vi "Data Array Tag.vi"(8 "error in (no error)":errorcluster, 11 "Node Ptr":T1 format="%.0x") -> (0 "error out":errorcluster)   [LabVIEW 2015, in "OPC UA Client System Explorer.lvlib"]
uses:
  OPC UA Client System Explorer.lvlib
  <vilib>/NI Veristand/Custom Device API/Custom Device Item Ref.ctl
  <vilib>/NI Veristand/Custom Device API/Custom Device API.lvlib
panel:
  out "Name":string
  in  "Header":cluster{"Section Name":string}={"Section Name"="Data Tag Settings"}
  in  "Description":string
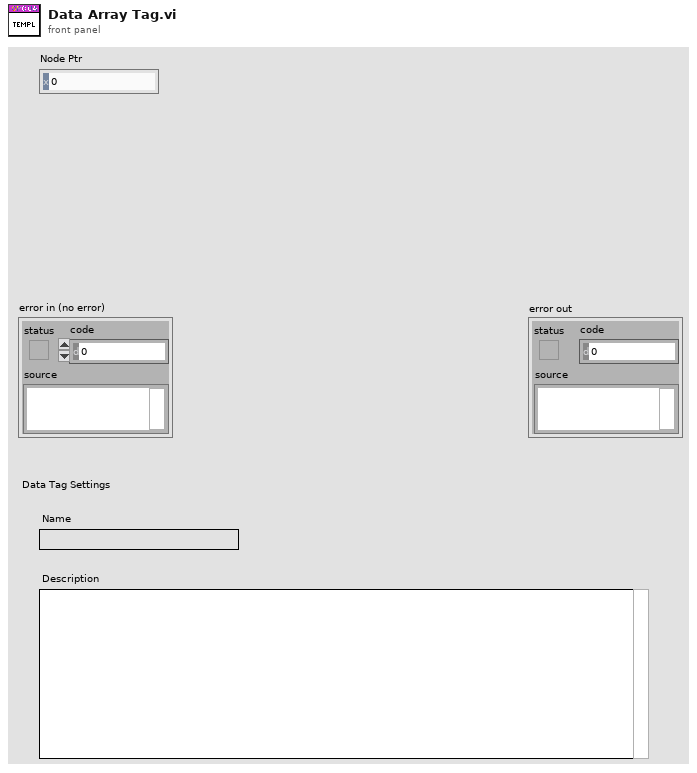
[diagram p1: front panel]
types:
  T1 = typedef "Custom Device API.lvlib/Custom Device Item Ref.ctl" = u64
  T2 = typedef "Custom Device API.lvlib/Custom Device Item Info.ctl" = cluster{"Name":string, "Is Channel":bool, "GUID":string, "Is Waveform":bool}
  T3 = typedef "Custom Device API.lvlib/Custom Device Commands.ctl" = enum16{"Default", "Item renamed", "Shutdown", "Dynamic button pressed"}
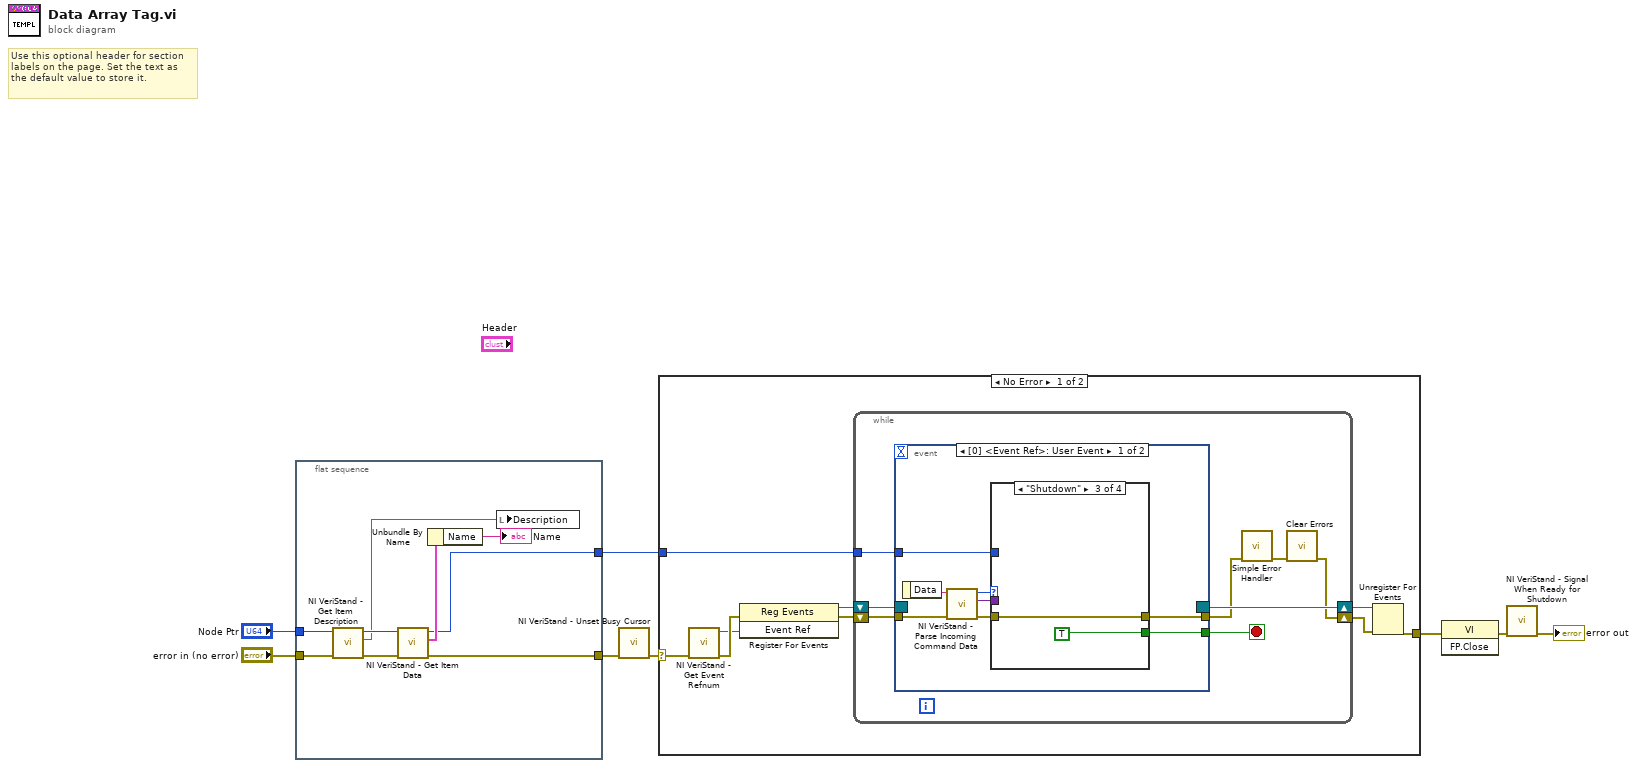
[diagram p0: block diagram]
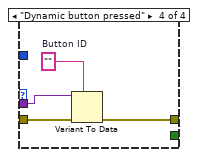
[diagram p4: hidden frame]
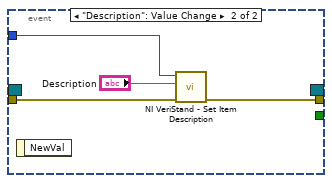
[diagram p5: hidden frame]
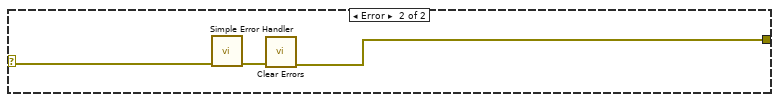
[diagram p6: hidden frame]
diagram:
  # "Use this optional header for section labels on the page. Set the text as the default value to store it."
  n1 = flat-sequence {
    tunnel: "Node Ptr" -> [w9]
    tunnel: "error in (no error)" -> [w10]
    tunnel: [w15] -> w3
    tunnel: [w13] -> w2
    frame #0 {
      n2 = call <vilib>:"NI VeriStand - Get Item Description.vi"("error in (no error)"=w10, "Item Ref in"=w9) -> ("error out"=w16:errorcluster, "Description"=w11:string, "Item Ref out"=w14:T1)  [unwired: 6 in, 1 out]
      n3 = call <vilib>:"NI VeriStand - Get Item Data.vi"("error in (no error)"=w16, "Item Ref in"=w14) -> ("error out"=w15:errorcluster, "Item Info"=w17:T2, "Item Ref out"=w13:T1)  [unwired: 7 out]
      n4 = Unbundle By Name(w17) -> ("Name"=→"Name":string)
      n5 = local write "Description"(w11) -> ()
    }
  }
  n6 = call <vilib>:"NI VeriStand - Unset Busy Cursor.vi"("error in (no error)"=w3) -> ("error out"=w5:errorcluster)  [unwired: 10 out]
  n7 = case shown="No Error" w5 {
    selector: w5 -> [w18 w57]
    tunnel: [w23 w55] -> w8
    tunnel: w2 -> [w19 _]
    frame No Error {
      n8 = call <vilib>:"NI VeriStand - Get Event Refnum.vi"("error in (no error)"=w18) -> ("error out"=w26:errorcluster, "Event Ref"=w22:refnum<user-event>)  [unwired: 9 out]
      n9 = register-events(error in=w26, w22) -> (reference out=w20:refnum<event-registration>, error out=w21:errorcluster)  [unwired: 1 in]
      n10 = while {
        tunnel: w19 -> [w30]
        shift-right: [w27] -> w24
        shift-left: w21 -> [w33]
        shift-right: [w34] -> w25
        shift-left: w20 -> [w32]
        stop <- w31 stop-if-true
        n11 = event shown="[0] <Event Ref>: User Event" {
          selector: w32 -> [_ _]
          dyn-events: [_ _] -> w34
          timeout: _ -> [_ _]
          tunnel: w33 -> [w42 w54]
          tunnel: [w38 _] -> w31
          tunnel: [w37 w52] -> w29
          tunnel: w30 -> [w36 w53]
          event User Event {
            n12 = event-data() -> ("Data"=w41:string)  [unwired: 1 out]
            n13 = call <vilib>:"NI VeriStand - Parse Incoming Command Data.vi"("error in (no error)"=w42, "Incoming data"=w41) -> ("error out"=w40:errorcluster, "Outgoing data"=w35:variant, "Action"=w39:T3)  [unwired: 7 out]
            n14 = case shown="\"Shutdown\"" w39 {
              tunnel: w40 -> [w43 w44 w45 w50]
              tunnel: [_ _ TRUE _] -> w38
              tunnel: [w43 w44 w45 w47] -> w37
              tunnel: w36 -> [_ _ _ _]
              tunnel: w35 -> [_ _ _ w49]
              frame "Default", Default {
              }
              frame "Item renamed" {
              }
              frame "Shutdown" {
              }
              frame "Dynamic button pressed" {
                w48 = ""  # Button ID
                n15 = Variant To Data(error in=w50, type=w48, Variant=w49) -> (error out=w47:errorcluster)  [unwired: 1 out]
              }
            }
          }
          event "Description": Value Change {
            n16 = event-data() -> ()  [unwired: 2 out]
            n17 = call <vilib>:"NI VeriStand - Set Item Description.vi"("error in (no error)"=w54, "Description"="Description", "Item Ref in"=w53) -> ("error out"=w52:errorcluster)  [unwired: 6 in, 2 out]
          }
        }
        n18 = call <vilib>:"Simple Error Handler.vi"("error in (no error)"=w29) -> ("error out"=w28:errorcluster)  [unwired: 1 in, 7 out]
        n19 = call <vilib>:"Clear Errors.vi"("error in (no error)"=w28) -> ("error out"=w27:errorcluster)  [unwired: 1 in, 5 out]
      }
      n20 = Unregister For Events(event registration refnum=w25, error in=w24) -> (error out=w23:errorcluster)
    }
    frame Error {
      n21 = call <vilib>:"Simple Error Handler.vi"("error in (no error)"=w57) -> ("error out"=w56:errorcluster)  [unwired: 1 in, 7 out]
      n22 = call <vilib>:"Clear Errors.vi"("error in (no error)"=w56) -> ("error out"=w55:errorcluster)  [unwired: 1 in, 5 out]
    }
  }
  n23 = invoke class="VI" method="FP.Close"(error in=w8) -> (error out=w7:errorcluster)  [unwired: 2 in, 2 out]
  n24 = call <vilib>:"NI VeriStand - Signal When Ready for Shutdown.vi"("error in (no error)"=w7) -> ("error out"=→"error out":errorcluster)  [unwired: 10 out]
